vi "CUBA.vi"() -> ()   [LabVIEW 2019]
uses:
  Control/Data Struct - Device Event Msg.ctl
  Control/Device Name.ctl
  Control/State - eFGV.ctl
panel:
  out "error out":errorcluster
  in  "Event Message":T1
  in  "OK Button":bool
  in  "stop":bool
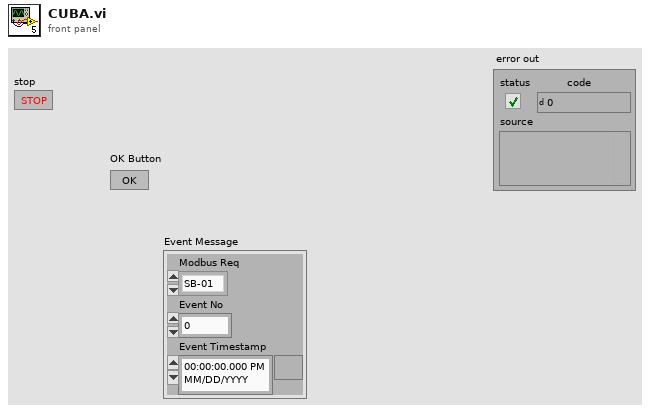
[diagram p1: front panel]
types:
  T1 = typedef "Data Struct - Device Event Msg.ctl" = cluster{"Modbus Req":T2, "Event No":u32, "Event Timestamp":timestamp}
  T2 = typedef "Device Name.ctl" = enum16{"SB-01", "SB-02", "SB-03", "SB-04", "STP-01", "STP-02", "STP-03", "STP-04", "BANK-01", "BANK-02", "BANK-03", "BANK-04", "SI-M-01", "SI-M-02", "SI-M-03", "SI-M-04", "PM-01"}
  T3 = typedef "State - eFGV.ctl" = enum16{"Init", "Read", "Write", "Close"}
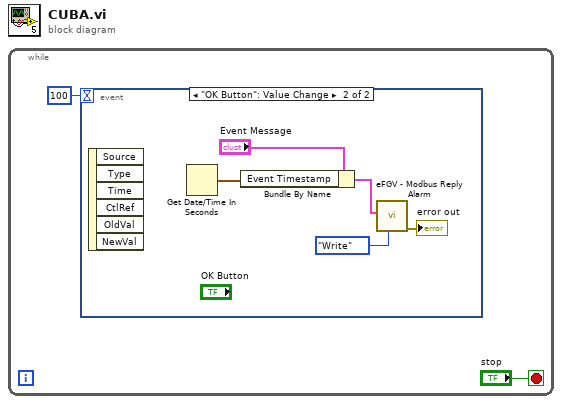
[diagram p0: block diagram]
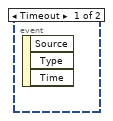
[diagram p2: hidden frame]
diagram:
  n1 = while {
    stop <- "stop" stop-if-true
    n2 = event shown="[1] \"OK Button\": Value Change" {
      selector: _ -> [_ _]
      dyn-events: _ -> [_ _]
      timeout: 100 -> [_ _]
      event Timeout {
        n3 = event-data() -> ()  [unwired: 1 in, 3 out]
      }
      event "OK Button": Value Change {
        n4 = event-data() -> ()  [unwired: 1 in, 6 out]
        n5 = Get Date/Time In Seconds() -> (seconds since 1Jan1904=w4:timestamp)
        n6 = Bundle By Name(cluster="Event Message", "Event Timestamp"=w4) -> (w5:T1)
        n7 = call "eFGV - Modbus Reply Alarm.vi"("State - eFGV"=State_-_eFGV."Write", "Event Message"=w5) -> ("error out"=→"error out":errorcluster)  [unwired: 8 in, 1 out]
      }
    }
  }
